vi "Configure Resistance Measurement (Aperture).vi"(6 "Aperture Type (1: Medium)":i32(ring)=1 items=["Short", "Medium", "Long"], 7 "Auto Resistance Aperture (T: Enable)":bool=TRUE, 8 "error in (no error)":errorcluster, 9 "Aperture Integration Time (0.002 s)":dbl=0.002, 10 "Channel (1: Channel 1)":i32(ring)=1 items=["Channel 1"=1, "Channel 2"=2], 11 "VISA resource name":refnum<visa-resource-name>) -> (0 "error out":errorcluster, 3 "VISA resource name out":refnum<visa-resource-name>)   [LabVIEW 2012, in "Keysight B2980 Series.lvlib"]
doc: "Configures the aperture settings for resistance measurement function.\n\n<b>Note(s):</b>\n(1) This VI is only applicable for model B2985A and B2987A.\n(2) Resistance measurement should be enabled from <b>Configure Measurement Function.vi</b>."
uses:
  Keysight B2980 Series.lvlib
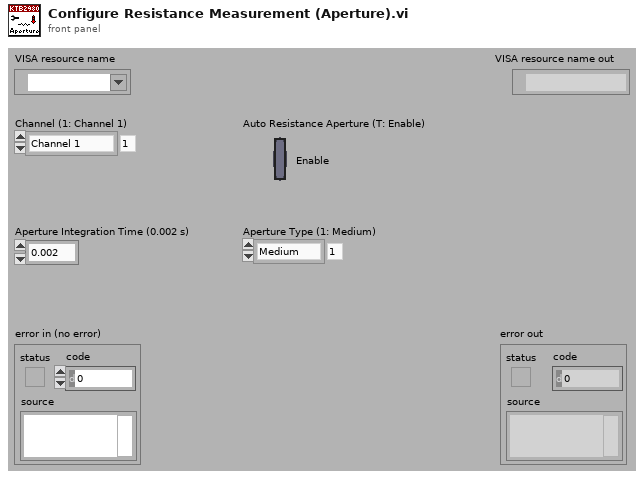
[diagram p1: front panel]
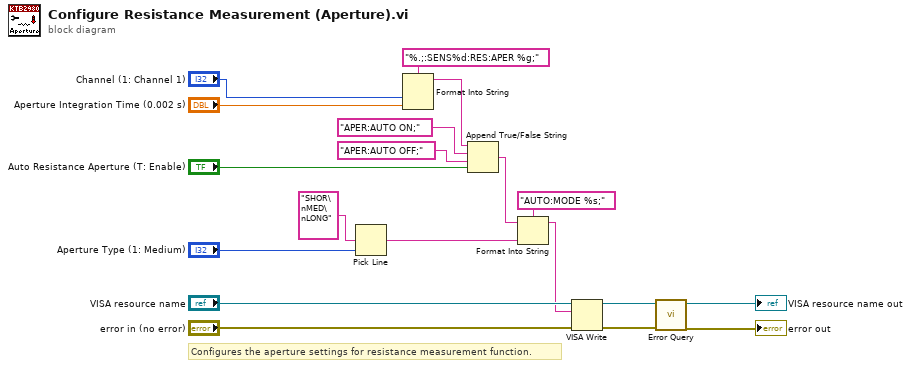
[diagram p0: block diagram]
diagram:
  # "Configures the aperture settings for resistance measurement function."
  n1 = Pick Line(multi-line string="SHOR\nMED\nLONG", line index="Aperture Type (1: Medium)") -> (output string=w7:string)  [unwired: 1 out]
  n2 = Format Into String(format string="%.;:SENS%d:RES:APER %g;", "Channel (1: Channel 1)", "Aperture Integration Time (0.002 s)") -> (resulting string=w10:string)  [unwired: 2 in, 1 out]
  n3 = Append True/False String(1:"Auto Resistance Aperture (T: Enable)", 2:"APER:AUTO OFF;", 3:"APER:AUTO ON;", 4:w10) -> (0:w6:string)
  n4 = Format Into String(format string="AUTO:MODE %s;", initial string=w6, w7) -> (resulting string=w1:string)  [unwired: 1 in, 1 out]
  n5 = VISA Write(VISA resource name="VISA resource name", write buffer=w1, error in (no error)="error in (no error)") -> (VISA resource name out=w17:refnum<visa-resource-name>, error out=w16:errorcluster)  [unwired: 1 out]
  n6 = call "Error Query.vi"("error in (no error)"=w16, "VISA resource name"=w17) -> ("error out"=→"error out":errorcluster, "VISA resource name out"=→"VISA resource name out":refnum<visa-resource-name>)  [unwired: 8 out]
